vi "getRfData.vi"(8 "error in (no error)":errorcluster, 11 "RfOutputData in":refnum<class "RfOutputData.lvclass">) -> (0 "error out":errorcluster, 2 "rfData":T1(array[cluster]), 3 "RfOutputData out":refnum<class "RfOutputData.lvclass">)   [LabVIEW 2011, in "DataMappers.lvlib" / "RfOutputData.lvclass"]
uses:
  RfOutputData.lvclass
  DatabaseHelpers/Database Objects/Channel/RfOutputChannel/RfOutputChannel.lvclass
  Scripting/ScriptingEvent/ScriptEvents/Rf Event/rf.lvclass
  Scripting/ScriptingEvent/ScriptEvents/RfRamp/RfRamp.lvclass
  RfOutputData.lvclass/RfOutputData.ctl
  DeviceData.lvclass
  DatabaseHelpers/Database Objects/device/device.lvclass
  Scripting/ScriptingEvent/ScriptEventList/ScriptEventList.lvclass
  Scripting/ScriptingEvent/ScriptEvent.lvclass
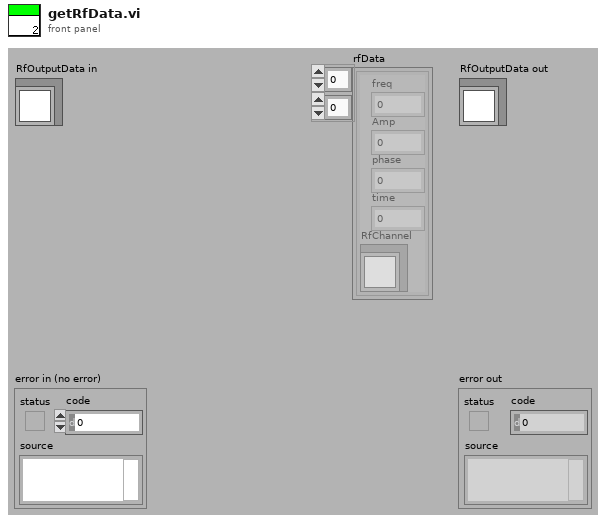
[diagram p1: front panel]
types:
  T1 = cluster{"freq":dbl, "Amp":dbl, "phase":dbl, "time":dbl, "RfChannel":refnum<class "RfOutputChannel.lvclass">}[][]
  T2 = cluster{"RfOutputChannel.lvclass":refnum<class "RfOutputChannel.lvclass">, "dataValue":dbl, "calibratedFreq":dbl, "calibratedPhase":dbl, "time":dbl}[]
  T3 = enum16{"changeValue", "pulse", "clock", "rampUp", "rampDown", "singleTone", "singleToneRamp", "playFile", "rf", "rfRamp", "delay"}
  T4 = cluster{"RfOutputChannel.lvclass":refnum<class "RfOutputChannel.lvclass">, "dataValue":dbl, "calibratedFreq":dbl, "calibratedPhase":dbl, "time":dbl}
  T5 = cluster{"RfOutputChannel":refnum<class "RfOutputChannel.lvclass">, "dataValue":dbl, "calibratedFreq":dbl, "calibratedPhase":dbl, "time":dbl}[]
  T6 = cluster{"RfOutputChannel.lvclass":refnum<class "RfOutputChannel.lvclass">, dbl[][]}[]
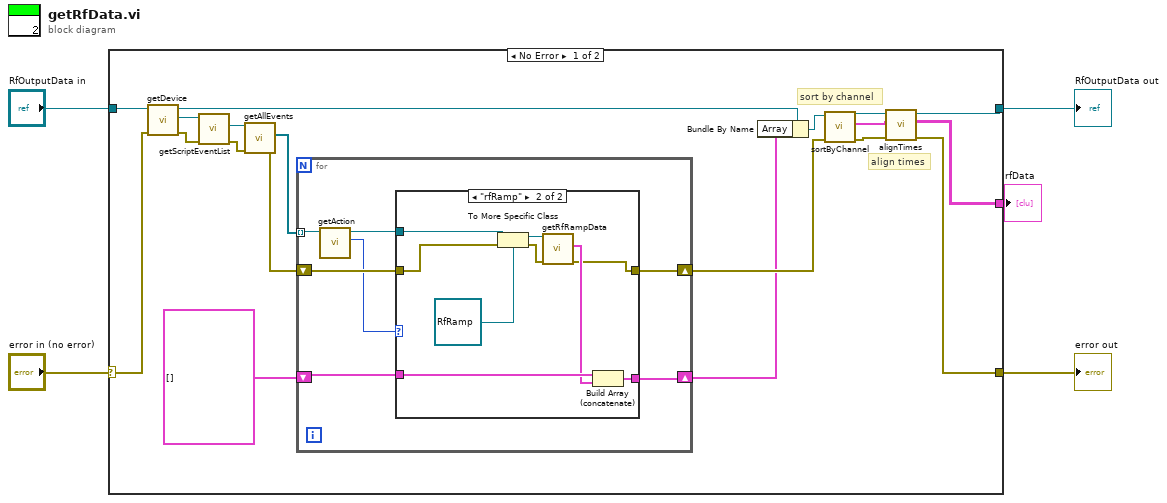
[diagram p0: block diagram]
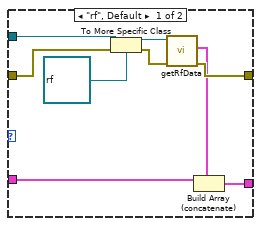
[diagram p2: hidden frame]
diagram:
  n1 = case shown="No Error" "error in (no error)" {
    selector: "error in (no error)" -> [w23 w51]
    tunnel: [w8 w51] -> w4
    tunnel: [w12 w50] -> w2
    tunnel: "RfOutputData in" -> [w24 w50]
    tunnel: [w10 _] -> w1
    frame No Error {
      # "align times"
      # "sort by channel"
      n2 = call "getDevice.vi"("error in (no error)"=w23, "DeviceData.lvclass in"=w24) -> ("error out"=w21:errorcluster, "device"=w22:refnum<class "device.lvclass">, "DeviceData.lvclass out"=w16:refnum<class "RfOutputData.lvclass">)  [unwired: 7 in]
      n3 = call "getScriptEventList.vi"("error in (no error)"=w21, "device.lvclass in"=w22) -> ("error out"=w19:errorcluster, "ScriptEventList"=w20:refnum<class "ScriptEventList.lvclass">)  [unwired: 7 in, 1 out]
      n4 = call "getAllEvents.vi"("error in (no error)"=w19, "ScriptEventList in"=w20) -> ("error out"=w17:errorcluster, "allScriptEvents"=w18:refnum<class "ScriptEvent.lvclass">[])  [unwired: 6 in, 2 out]
      n5 = for {
        tunnel: w18 -> [w29] mode=indexing
        shift-right: [w31] -> w14
        shift-left: w17 -> [w30]
        shift-right: [w25] -> w6
        shift-left: T2 [] -> [w26]
        n6 = call "getAction.vi"("ScriptEvent.lvclass in"=w29) -> ("action"=w27:T3, "ScriptEvent.lvclass out"=w28:refnum<class "ScriptEvent.lvclass">)  [unwired: 8 in, 1 out]
        n7 = case shown="\"rfRamp\"" w27 {
          tunnel: [w37 w41] -> w31
          tunnel: w30 -> [w36 w49]
          tunnel: w28 -> [w35 w48]
          tunnel: w26 -> [w34 w44]
          tunnel: [w32 w43] -> w25
          frame "rf", Default {
            n8 = To More Specific Class(target class=refnum<class "rf.lvclass"> refnum ("rf in"), reference=w35, error in=w36) -> (specific class reference=w38:refnum<class "rf.lvclass">, error out=w40:errorcluster)
            n9 = call "getRfData.vi"("error in (no error)"=w40, "rf in"=w38) -> ("error out"=w37:errorcluster, "data"=w33:T4)  [unwired: 7 in, 1 out]
            n10 = Build Array (concatenate)(w34, w33) -> (w32:T2)
          }
          frame "rfRamp" {
            n11 = To More Specific Class(target class=refnum<class "RfRamp.lvclass"> refnum ("Tools.lvlib:Scripting.lvlib:RfRamp.lvclass"), reference=w48, error in=w49) -> (specific class reference=w46:refnum<class "RfRamp.lvclass">, error out=w45:errorcluster)
            n12 = call "getRfRampData.vi"("error in (no error)"=w45, "RfRamp in"=w46) -> ("error out"=w41:errorcluster, "Array"=w42:T5)  [unwired: 7 in, 1 out]
            n13 = Build Array (concatenate)(w44, w42) -> (w43:T5)
          }
        }
      }
      n14 = Bundle By Name(cluster=w16, "Array"=w6) -> (w15:refnum<class "RfOutputData.lvclass">)
      n15 = call "sortByChannel.vi"("error in (no error)"=w14, "RfOutputData in"=w15) -> ("error out"=w9:errorcluster, "sortedData"=w11:T6, "RfOutputData out"=w13:refnum<class "RfOutputData.lvclass">)  [unwired: 7 in]
      n16 = call "alignTimes.vi"("error in (no error)"=w9, "sortedData"=w11, "RfOutputData in"=w13) -> ("error out"=w8:errorcluster, "rfData"=w10:T1, "RfOutputData out"=w12:refnum<class "RfOutputData.lvclass">)  [unwired: 6 in]
    }
    frame Error {
    }
  }
  "error out" <- w4
  "RfOutputData out" <- w2
  "rfData" <- w1
